vi "Find String with Start and Option.vi"(7 "options":i32(ring) items=["None"=0, "WholeWord"=2, "MatchCase"=4, "NoHighlight"=8, "Reverse"=16], 8 "error in (no error)":errorcluster caption="错误输入（无错误）", 9 "start":i32, 10 "str":string, 11 "RichText 输入":refnum<class "RichText.lvclass"> caption="DNL_LabVIEW Object in") -> (0 "error out":errorcluster caption="错误输出", 2 "Find":i32, 3 "RichText 输出":refnum<class "RichText.lvclass"> caption="DNL_LabVIEW Object out")   [LabVIEW 2012, in "RichText.lvclass"]
uses:
  RichText.lvclass
  RichText.lvclass/RichText.ctl
  System.Windows.Forms
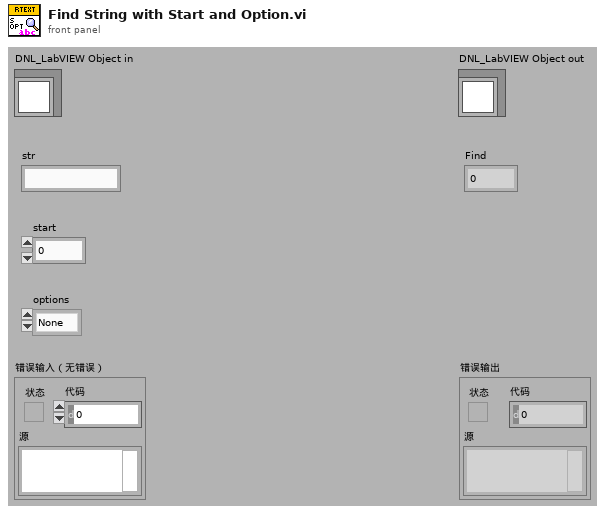
[diagram p1: front panel]
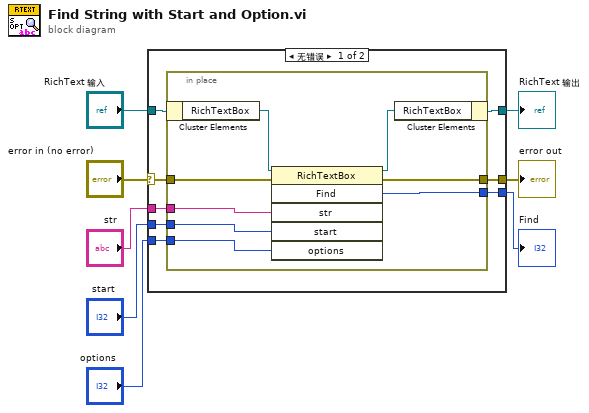
[diagram p0: block diagram]
diagram:
  n1 = case shown="无错误" "error in (no error)" {
    selector: "error in (no error)" -> [w10 w26]
    tunnel: [w9 w26] -> w7
    tunnel: [w14 w25] -> w5
    tunnel: "RichText 输入" -> [w16 w25]
    tunnel: [w15 _] -> w4
    tunnel: "str" -> [w13 _]
    tunnel: "start" -> [w12 _]
    tunnel: "options" -> [w11 _]
    frame No Error {
      n2 = in-place {
        in-place-border: [w22] -> w15
        in-place-border: w13 -> [w21]
        in-place-border: w12 -> [w20]
        in-place-border: w11 -> [w19]
        in-place-border: w10 -> [w18]
        in-place-border: [w17] -> w9
        n3 = in-place-cluster #1(w16) -> ("RichTextBox"=w24:refnum<k24>)
        n4 = invoke class="RichTextBox" method="Find"(reference=w24, error in=w18, "str"=w21, "start"=w20, "options"=w19) -> (reference out=w23:refnum<k24>, error out=w17:errorcluster, "Find"=w22:i32)  [unwired: 1 in, 3 out]
        n5 = in-place-cluster #1("RichTextBox"=w23) -> (w14:refnum<class "RichText.lvclass">)
      }
    }
    frame Error {
    }
  }
  "error out" <- w7
  "RichText 输出" <- w5
  "Find" <- w4
